vi "Handle Error.vi"(8 "error in (no error)":errorcluster, 11 "PLC_Module in":refnum<class "PLC_Module.lvclass">) -> (0 "error out":errorcluster, 2 "stop actor?":bool=TRUE, 3 "PLC_Module out":refnum<class "PLC_Module.lvclass">)   [LabVIEW 2025, in "PLC_Module.lvlib" / "PLC_Module.lvclass"]
doc: "<p>(<strong>Filename</strong>: <span class=\"dnl\">Actor Framework.lvlib:Actor.lvclass:Handle Error.vi</span>)</p>\n<p>Defines how the actor handles an error that occurred while processing a message. By default, this method does nothing except stop the actor.</p>"
uses:
  PLC_Module.lvclass
  Module/Module/Module/Module.lvclass
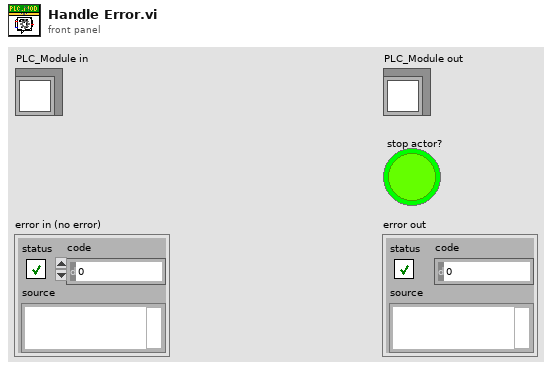
[diagram p1: front panel]
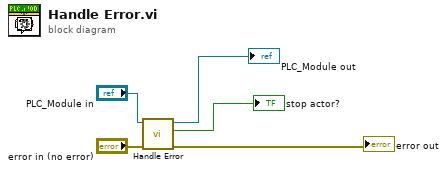
[diagram p0: block diagram]
diagram:
  n1 = call-parent "Handle Error.vi"("error in (no error)"="error in (no error)", "Actor in"="PLC_Module in") -> ("error out"=→"error out":errorcluster, "stop actor?"=→"stop actor?":bool, "Actor out"=→"PLC_Module out":refnum<class "PLC_Module.lvclass">)  [unwired: 7 in]
